vi "Process.vi"(2 "shared":refnum<class "niUSRP Tx Core v1 FPGA.lvclass">) -> ()   [LabVIEW 2025, in "niUSRP Tx Core v1 FPGA.lvclass"]
doc: "this VI calls the process VIs for Alignment, Routing, and LED Status."
uses:
  niUSRP Tx Core v1 FPGA.lvclass
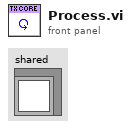
[diagram p1: front panel]
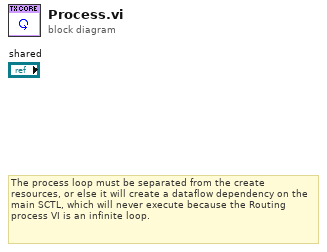
[diagram p0: block diagram]
diagram:
  # "The process loop must be separated from the create resources, or else it will create a dataflow dependency on the main SCTL, which will never execute because the Routing process VI is an infinite loop."
